vi "XML.Limits.Load.vi"(8 "error in":errorcluster, 10 "Limits file path":path) -> (0 "error out":errorcluster, 1 "StepIDs":string[](array[string]), 2 "Step.Limits":T1[](array[typedef]), 3 "DateOfCreate":string, 4 "MainSeq":string, 5 "FileVersion":string, 6 "StepRoots":string[](array[string]))   [LabVIEW 2019, in "Tools.lvlib"]
uses:
  Tools.lvlib
  TestStand/Import limits/ExecutingSeqNoSave/controls/TS.Step.LoadSeqLimits.StepLimits.ctl
  LibXML/LibXML.lvlib
panel:
  out "Duration":u32
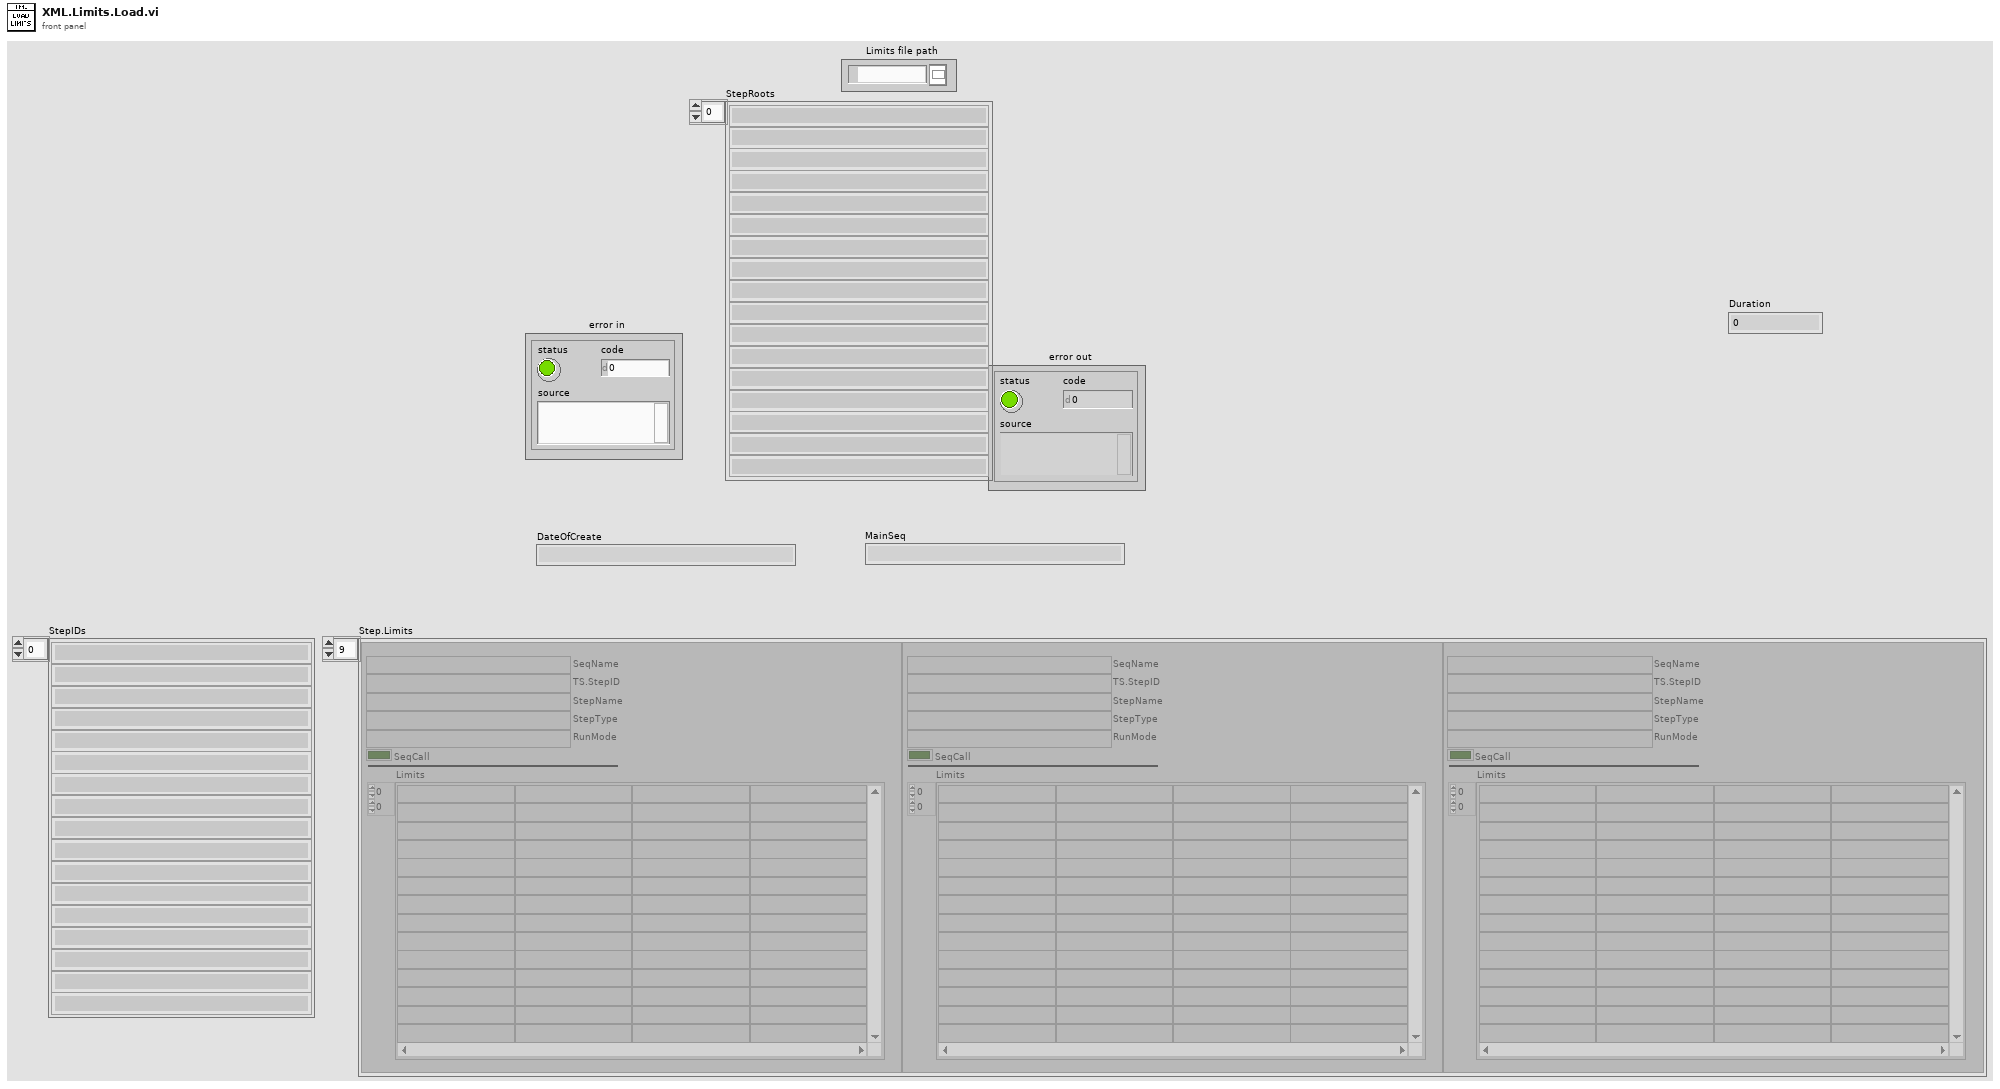
[diagram p1: front panel]
types:
  T1 = typedef "TS.Step.LoadSeqLimits.StepLimits.ctl" = cluster{"SeqName":string, "TS.StepID":string, "StepName":string, "StepType":string, "RunMode":string, "SeqCall":bool, "Limits":string[][]}
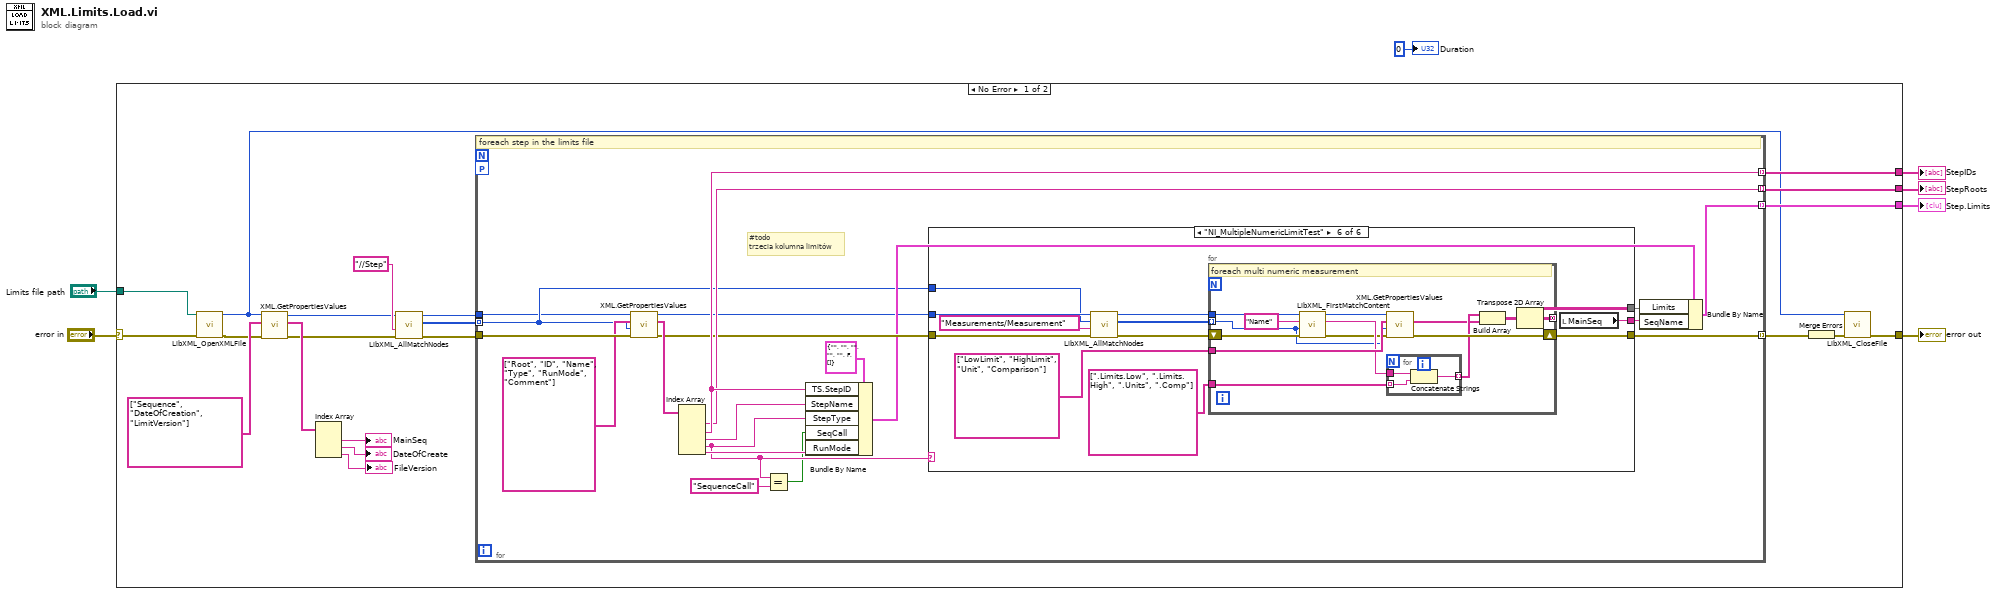
[diagram p0: block diagram]
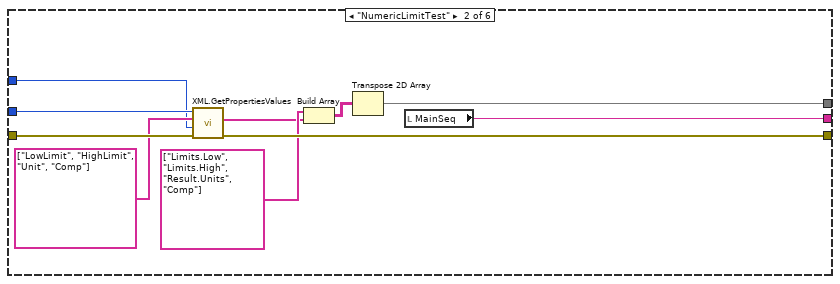
[diagram p3: hidden frame]
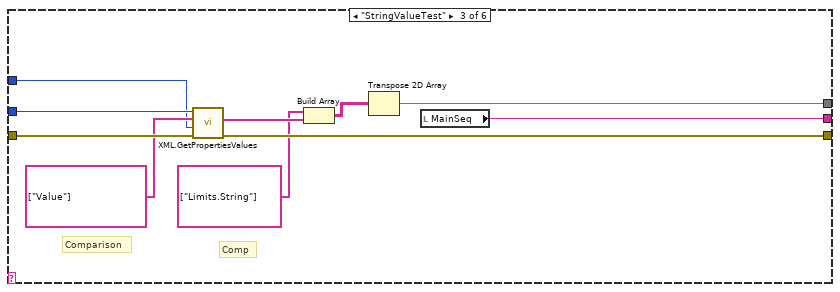
[diagram p4: hidden frame]
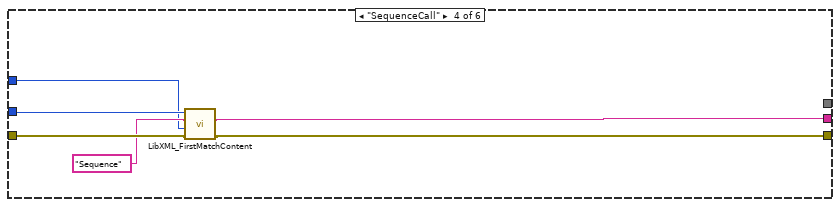
[diagram p5: hidden frame]
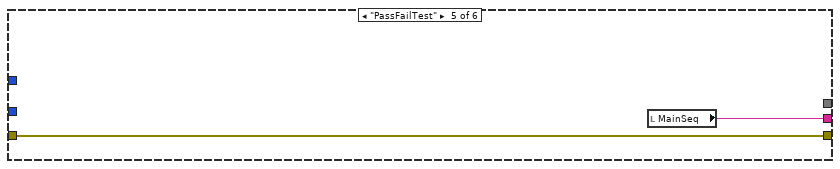
[diagram p6: hidden frame]
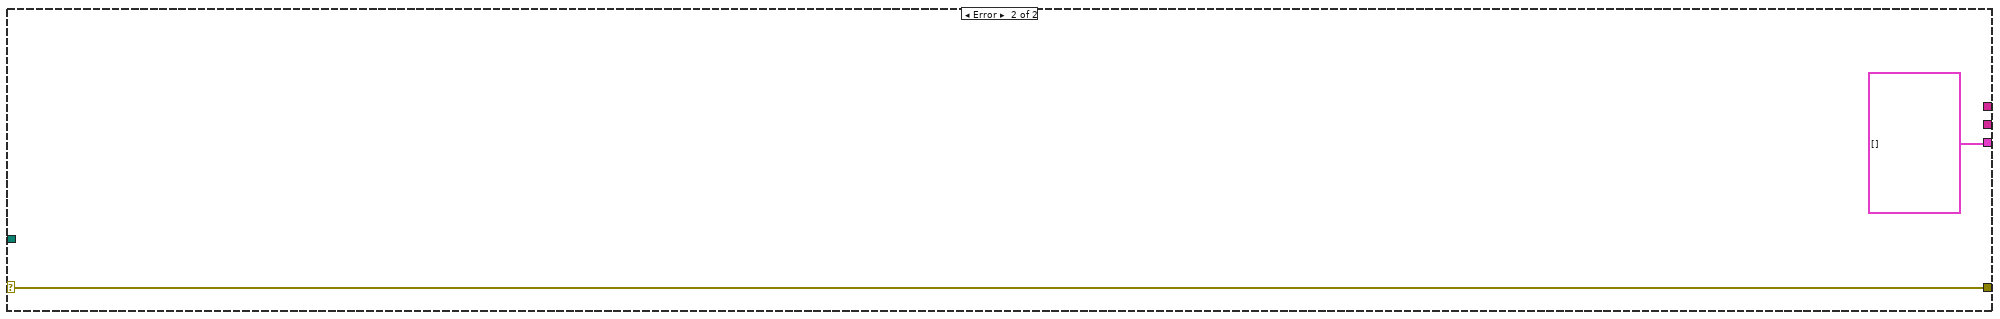
[diagram p7: hidden frame]
diagram:
  n1 = case shown="No Error" "error in" {
    selector: "error in" -> [w9 w108]
    tunnel: [w8 w108] -> w7
    tunnel: [w20 T1[] []] -> w3
    tunnel: [w23 _] -> w1
    tunnel: "Limits file path" -> [w19 _]
    tunnel: [w22 _] -> w2
    frame No Error {
      n2 = call "LibXML_OpenXMLFile.vi"("error in"=w9, "file path"=w19) -> ("error out"=w18:errorcluster, "doc"=w13:u32)  [unwired: 7 in, 1 out]
      n3 = call "XML.GetPropertiesValues.vi"("error in"=w18, "property names"=string[] ["Sequence", "DateOfCreation", "LimitVersion"], "XML ref in"=w13) -> ("error out"=w16:errorcluster, "property values"=w27:string[], "XML ref out"=w10:u32)  [unwired: 6 in]
      n4 = Index Array(array=w27) -> (element #1=→"MainSeq":string, element #2=→"DateOfCreate":string, element #3=→"FileVersion":string)  [unwired: 3 in]
      n5 = call "LibXML_AllMatchNodes.vi"("error in"=w16, "XPath"="//Step" ("XPath expression"), "doc"=w10) -> ("error out"=w15:errorcluster, "Matched Nodes"=w14:u32[], "doc out"=w11:u32)  [unwired: 6 in]
      n6 = for {
        tunnel: w14 -> [w30] mode=indexing
        tunnel: [w40] -> w23 mode=indexing
        tunnel: [w39] -> w22 mode=indexing
        tunnel: [w33] -> w20 mode=indexing
        tunnel: w15 -> [w38]
        tunnel: [w31] -> w21 mode=indexing
        workers-P: _ -> [_]
        tunnel: w11 -> [w29]
        # "#todo\ntrzecia kolumna limitów"
        # "foreach step in the limits file"
        n7 = call "XML.GetPropertiesValues.vi"("error in"=w38, "rootnode (root of doc)"=w30, "property names"=string[] ["Root", "ID", "Name", "Type", "RunMode", "Comment"], "XML ref in"=w29) -> ("error out"=w35:errorcluster, "property values"=w37:string[], "XML ref out"=w32:u32)  [unwired: 5 in]
        n8 = Index Array(array=w37) -> (element #1=w39:string, element #2=w40:string, element #3=w47:string, element #4=w44:string, element #5=w46:string)  [unwired: 5 in]
        n9 = Equal?(x=w44, y="SequenceCall") -> (x = y?=w41:bool)
        n10 = Bundle By Name(cluster=T1 {"SeqName"="", "TS.StepID"="", "StepName"="", "StepType"="", "RunMode"="", "SeqCall"=FALSE, "Limits"=[]} ("Step limits"), "TS.StepID"=w40, "StepName"=w47, "StepType"=w44, "SeqCall"=w41, "RunMode"=w46) -> (w34:T1)
        n11 = case shown="\"NI_MultipleNumericLimitTest\"" w44 {
          tunnel: w32 -> [_ w58 w68 w72 _ w80]
          tunnel: [_ w51 w61 _ _ w87] -> w43
          tunnel: [_ w59 w69 w71 w77 w86] -> w42
          tunnel: w35 -> [w49 w57 w67 w75 w76 w84]
          tunnel: [w49 w56 w66 w74 w76 w85] -> w31
          tunnel: w30 -> [_ w50 w60 w70 _ w79]
          frame Default {
          }
          frame "NumericLimitTest" {
            n12 = call "XML.GetPropertiesValues.vi"("error in"=w57, "rootnode (root of doc)"=w50, "property names"=string[] ["LowLimit", "HighLimit", "Unit", "Comp"], "XML ref in"=w58) -> ("error out"=w56:errorcluster, "property values"=w53:string[])  [unwired: 5 in, 1 out]
            n13 = Build Array(string[] ["Limits.Low", "Limits.High", "Result.Units", "Comp"], w53) -> (w52:string[][])
            n14 = Transpose 2D Array(2D array=w52) -> (transposed array=w51:string[][])
            n15 = local read "MainSeq"() -> (w59:string)
          }
          frame "StringValueTest" {
            # "Comparison"
            # "Comp"
            n16 = call "XML.GetPropertiesValues.vi"("error in"=w67, "rootnode (root of doc)"=w60, "property names"=string[] ["Value"], "XML ref in"=w68) -> ("error out"=w66:errorcluster, "property values"=w65:string[])  [unwired: 5 in, 1 out]
            n17 = Build Array(string[] ["Limits.String"], w65) -> (w64:string[][])
            n18 = Transpose 2D Array(2D array=w64) -> (transposed array=w61:string[][])
            n19 = local read "MainSeq"() -> (w69:string)
          }
          frame "SequenceCall" {
            n20 = call "LibXML_FirstMatchContent.vi"("error in"=w75, "rootnode (root of doc)"=w70, "xpathexpr"="Sequence" ("XPath expression"), "doc in"=w72) -> ("error out"=w74:errorcluster, "content"=w71:string)  [unwired: 5 in, 1 out]
          }
          frame "PassFailTest" {
            n21 = local read "MainSeq"() -> (w77:string)
          }
          frame "NI_MultipleNumericLimitTest" {
            n22 = call "LibXML_AllMatchNodes.vi"("error in"=w84, "XPath"="Measurements/Measurement" ("XPath expression"), "root node"=w79, "doc"=w80) -> ("error out"=w83:errorcluster, "Matched Nodes"=w82:u32[], "doc out"=w78:u32)  [unwired: 5 in]
            n23 = for {
              tunnel: w82 -> [w90] mode=indexing
              tunnel: string[] ["LowLimit", "HighLimit", "Unit", "Comparison"] -> [w102]
              tunnel: string[] [".Limits.Low", ".Limits.High", ".Units", ".Comp"] -> [w103]
              tunnel: [w97] -> w87 mode=concatenating
              shift-right: [w101] -> w85
              shift-left: w83 -> [w94]
              tunnel: w78 -> [w91]
              # "foreach multi numeric measurement"
              n24 = call "LibXML_FirstMatchContent.vi"("error in"=w94, "rootnode (root of doc)"=w90, "xpathexpr"="Name" ("XPath expression"), "doc in"=w91) -> ("error out"=w95:errorcluster, "content"=w96:string, "doc copy out"=w92:u32)  [unwired: 5 in]
              n25 = call "XML.GetPropertiesValues.vi"("error in"=w95, "rootnode (root of doc)"=w90, "property names"=w102, "XML ref in"=w92) -> ("error out"=w101:errorcluster, "property values"=w99:string[])  [unwired: 5 in, 1 out]
              n26 = for {
                tunnel: w103 -> [w106] mode=indexing
                tunnel: w96 -> [w105]
                tunnel: [w104] -> w100 mode=indexing
                n27 = Concatenate Strings(w105, w106) -> (w104:string)
              }
              n28 = Build Array(w100, w99) -> (w98:string[][])
              n29 = Transpose 2D Array(2D array=w98) -> (transposed array=w97:string[][])
            }
            n30 = local read "MainSeq"() -> (w86:string)
          }
        }
        n31 = Bundle By Name(cluster=w34, "Limits"=w43, "SeqName"=w42) -> (w33:T1)
      }
      n32 = Merge Errors(w21) -> (w12:errorcluster)
      n33 = call "LibXML_CloseFile.vi"("error in"=w12, "doc"=w13) -> ("error out"=w8:errorcluster)  [unwired: 9 in]
    }
    frame Error {
    }
  }
  "error out" <- w7
  "StepIDs" <- w1
  "Step.Limits" <- w3
  "StepRoots" <- w2
  "Duration" <- u32 0 ("Duration")
